vi "Select Desired Excel Worksheets.vi"(8 "error in (no error)":errorcluster, 11 "ExcelRefs in":T1) -> (0 "error out":errorcluster, 1 "Cancelled":bool, 2 "Selected Worksheets":string[](array[string]), 3 "ExcelRefs dup":T1)   [LabVIEW 2011]
uses:
  Controls/Excel Refs.ctl
  <userlib>/_OpenG.lib/array/array.llb/Conditional Auto-Indexing Tunnel (I32)__ogtk.vi
  <userlib>/_OpenG.lib/array/array.llb/Delete Elements from 1D Array (String)__ogtk.vi
panel:
  in  "Result Filter":string="_TestVec"
  in  "Cancel":bool
  in  "Import":bool
  in  "Add":bool
  in  "Remove":bool
  in  "ToImport":i32[](listbox) caption="Worksheets to import"
  in  "Avail":i32[](listbox) caption="Available worksheets"
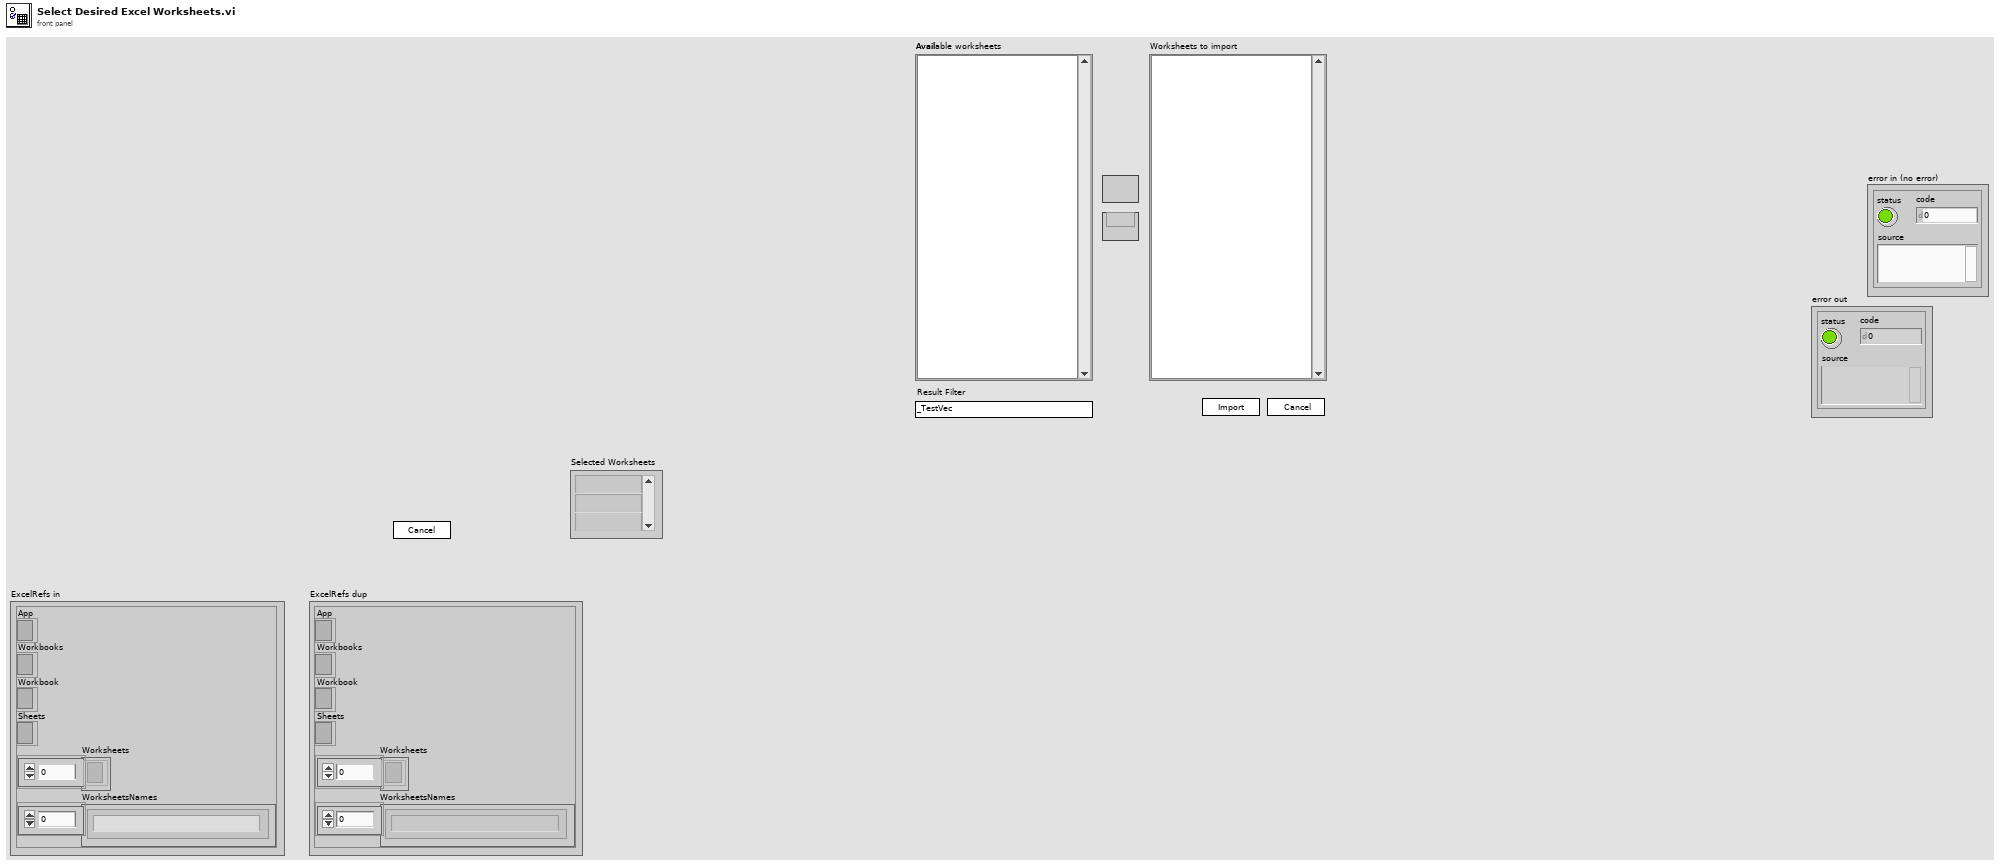
[diagram p1: front panel]
types:
  T1 = typedef "Excel Refs.ctl" = cluster{"App":refnum<k7>, "Workbooks":refnum<k7>, "Workbook":refnum<k7>, "Sheets":refnum<k7>, "Worksheets":refnum<k7>[], "WorksheetsNames":string[]}
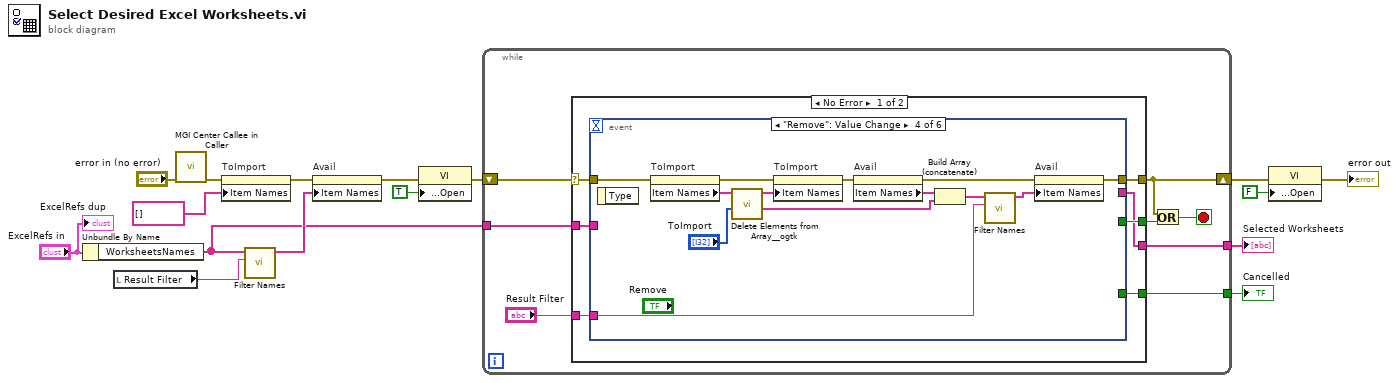
[diagram p0: block diagram]
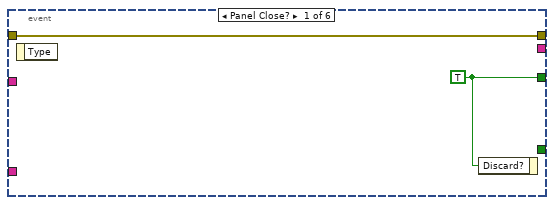
[diagram p2: hidden frame]
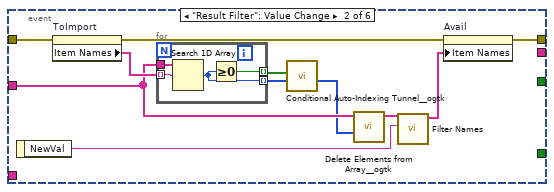
[diagram p3: hidden frame]
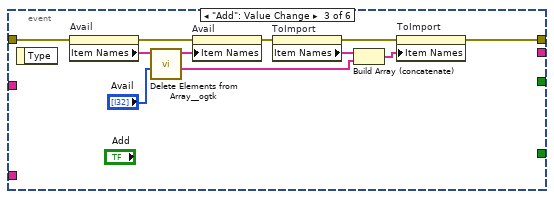
[diagram p4: hidden frame]
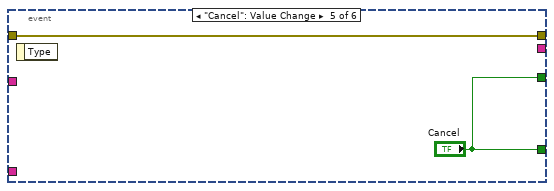
[diagram p5: hidden frame]
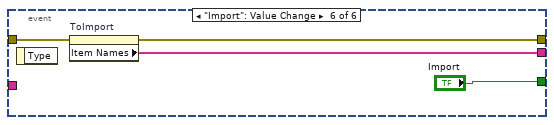
[diagram p6: hidden frame]
diagram:
  n1 = Unbundle By Name("ExcelRefs in") -> ("WorksheetsNames"=w4:string[])
  n2 = local read "Result Filter"() -> (w6:string)
  n3 = call <userlib>:"MGI Center Callee in Caller.vi"("Error In"="error in (no error)") -> ("Error Out"=w3:errorcluster)  [unwired: 10 in]
  n4 = property on="ToImport" class="LstBox (strict)"(error in=w3, "Item Names"=string[] []) -> (error out=w2:errorcluster)  [unwired: 1 in, 1 out]
  n5 = call "Filter Names.vi"("Result Filter"=w6, "WorksheetsNames"=w4) -> ("Filtered"=w5:string[])  [unwired: 9 in]
  n6 = property on="Avail" class="LstBox (strict)"(error in=w2, "Item Names"=w5) -> (error out=w8:errorcluster)  [unwired: 1 in, 1 out]
  n7 = property on="Property Node" class="VI"(error in=w8, "Front Panel.Open"=TRUE ("Front Panel Window:Open")) -> (error out=w12:errorcluster)  [unwired: 1 in, 1 out]
  n8 = while {
    shift-right: [w21] -> w11
    shift-left: w12 -> [w22]
    tunnel: [w20] -> w10
    tunnel: [w19] -> w9
    tunnel: w4 -> [w17]
    stop <- w23 stop-if-true
    n9 = case shown="No Error" w22 {
      selector: w22 -> [w30 w79]
      tunnel: [w28 _] -> w24
      tunnel: [w31 w79] -> w21
      tunnel: [w29 _] -> w20
      tunnel: [w27 _] -> w19
      tunnel: "Result Filter" -> [w26 _]
      tunnel: w17 -> [w25 _]
      frame No Error {
        n10 = event shown="[3] \"Remove\": Value Change" {
          selector: _ -> [_ _ _ _ _ _]
          dyn-events: _ -> [_ _ _ _ _ _]
          timeout: _ -> [_ _ _ _ _ _]
          tunnel: [w32 w43 w56 w72 w73 w77] -> w31
          tunnel: w30 -> [w32 w41 w59 w67 w73 w78]
          tunnel: [_ _ _ _ "Cancel" _] -> w29
          tunnel: [w33 _ _ _ "Cancel" "Import"] -> w28
          tunnel: [_ _ _ _ _ w75] -> w27
          tunnel: w26 -> [_ _ _ w60 _ _]
          tunnel: w25 -> [_ w39 _ _ _ _]
          event Panel Close? {
            w33 = TRUE ("Discard?")
            n11 = event-data() -> ()  [unwired: 1 in, 1 out]
            n12 = event-data("Discard?"=w33) -> ()  [unwired: 1 in, 1 out]
          }
          event "Result Filter": Value Change {
            n13 = event-data() -> ("NewVal"=w42:string)  [unwired: 1 in]
            n14 = property on="ToImport" class="LstBox (strict)"(error in=w41) -> (error out=w38:errorcluster, "Item Names"=w40:string[])  [unwired: 1 in, 1 out]
            n15 = for {
              tunnel: w39 -> [w48]
              tunnel: w40 -> [w47] mode=indexing
              tunnel: [w46] -> w36 mode=indexing
              tunnel: [w45] -> w35 mode=indexing
              n16 = Search 1D Array(1D array=w48, element=w47) -> (index of element=w45:i32)  [unwired: 1 in]
              n17 = Greater Or Equal To 0?(x=w45) -> (x >= 0?=w46:bool)
            }
            n18 = call-poly <userlib>:"Conditional Auto-Indexing Tunnel__ogtk.vi"("Array in"=w35, "Elements to keep"=w36) -> ("Filtered Array out"=w34:i32[])  [unwired: 5 in]
            n19 = call-poly <userlib>:"Delete Elements from Array__ogtk.vi"("indices"=w34, "array"=w39) -> ("array w/ subset deleted"=w37:string[])  [unwired: 8 in, 1 out]
            n20 = call "Filter Names.vi"("Result Filter"=w42, "WorksheetsNames"=w37) -> ("Filtered"=w44:string[])  [unwired: 9 in]
            n21 = property on="Avail" class="LstBox (strict)"(error in=w38, "Item Names"=w44) -> (error out=w43:errorcluster)  [unwired: 1 in, 1 out]
          }
          event "Add": Value Change {
            n22 = event-data() -> ()  [unwired: 1 in, 1 out]
            n23 = property on="Avail" class="LstBox (strict)"(error in=w59) -> (error out=w50:errorcluster, "Item Names"=w58:string[])  [unwired: 1 in, 1 out]
            n24 = call-poly <userlib>:"Delete Elements from Array__ogtk.vi"("indices"="Avail", "array"=w58) -> ("deleted elements"=w53:string[], "array w/ subset deleted"=w49:string[])  [unwired: 8 in]
            n25 = property on="Avail" class="LstBox (strict)"(error in=w50, "Item Names"=w49) -> (error out=w51:errorcluster)  [unwired: 1 in, 1 out]
            n26 = property on="ToImport" class="LstBox (strict)"(error in=w51) -> (error out=w55:errorcluster, "Item Names"=w54:string[])  [unwired: 1 in, 1 out]
            n27 = Build Array (concatenate)(w54, w53) -> (w52:string[])
            n28 = property on="ToImport" class="LstBox (strict)"(error in=w55, "Item Names"=w52) -> (error out=w56:errorcluster)  [unwired: 1 in, 1 out]
          }
          event "Remove": Value Change {
            n29 = event-data() -> ()  [unwired: 1 in, 1 out]
            n30 = property on="ToImport" class="LstBox (strict)"(error in=w67) -> (error out=w68:errorcluster, "Item Names"=w66:string[])  [unwired: 1 in, 1 out]
            n31 = call-poly <userlib>:"Delete Elements from Array__ogtk.vi"("indices"="ToImport", "array"=w66) -> ("deleted elements"=w64:string[], "array w/ subset deleted"=w65:string[])  [unwired: 8 in]
            n32 = property on="ToImport" class="LstBox (strict)"(error in=w68, "Item Names"=w65) -> (error out=w69:errorcluster)  [unwired: 1 in, 1 out]
            n33 = property on="Avail" class="LstBox (strict)"(error in=w69) -> (error out=w71:errorcluster, "Item Names"=w70:string[])  [unwired: 1 in, 1 out]
            n34 = Build Array (concatenate)(w70, w64) -> (w62:string[])
            n35 = call "Filter Names.vi"("Result Filter"=w60, "WorksheetsNames"=w62) -> ("Filtered"=w61:string[])  [unwired: 9 in]
            n36 = property on="Avail" class="LstBox (strict)"(error in=w71, "Item Names"=w61) -> (error out=w72:errorcluster)  [unwired: 1 in, 1 out]
          }
          event "Cancel": Value Change {
            n37 = event-data() -> ()  [unwired: 1 in, 1 out]
          }
          event "Import": Value Change {
            n38 = event-data() -> ()  [unwired: 1 in, 1 out]
            n39 = property on="ToImport" class="LstBox (strict)"(error in=w78) -> (error out=w77:errorcluster, "Item Names"=w75:string[])  [unwired: 1 in, 1 out]
          }
        }
      }
      frame Error {
      }
    }
    n40 = Or(x=w21, y=w24) -> (x .or. y?=w23:bool)
  }
  "Selected Worksheets" <- w9
  "Cancelled" <- w10
  n41 = property on="Property Node" class="VI"(error in=w11, "Front Panel.Open"=FALSE ("Front Panel Window:Open")) -> (error out=→"error out":errorcluster)  [unwired: 1 in, 1 out]
  "ExcelRefs dup" <- "ExcelRefs in"
